vi "Read row.vi"(8 "error in (no error)":errorcluster, 11 "CellValueChanged in":refnum<class "CellDirtyStateChanged.lvclass">) -> (0 "error out":errorcluster, 2 "row":i32, 3 "CellValueChanged out":refnum<class "CellDirtyStateChanged.lvclass">)   [LabVIEW 2013, in "DataGrid.lvlib" / "CellDirtyStateChanged.lvclass"]
uses:
  CellDirtyStateChanged.lvclass
  CellDirtyStateChanged.lvclass/CellDirtyStateChanged.ctl
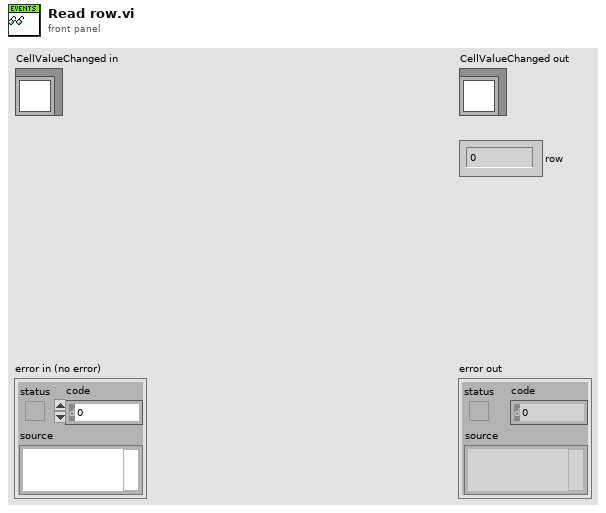
[diagram p1: front panel]
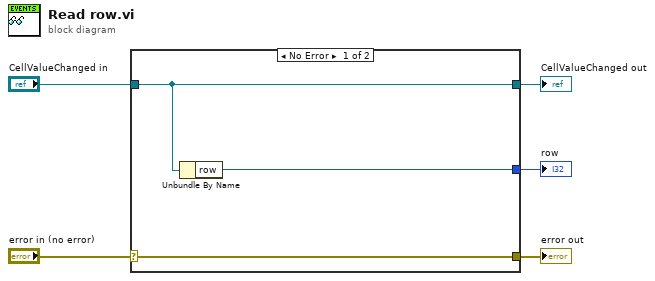
[diagram p0: block diagram]
diagram:
  n1 = case shown="No Error" "error in (no error)" {
    selector: "error in (no error)" -> [w8 w9]
    tunnel: [w8 w9] -> w4
    tunnel: [w7 w10] -> w2
    tunnel: "CellValueChanged in" -> [w7 w10]
    tunnel: [w6 _] -> w1
    frame No Error {
      n2 = Unbundle By Name(w7) -> ("row"=w6:i32)
    }
    frame Error {
    }
  }
  "error out" <- w4
  "CellValueChanged out" <- w2
  "row" <- w1
